vi "Check For Errors.vi"(8 "error in":errorcluster, 11 "Engine in":refnum<class "Engine.lvclass">) -> (0 "error out":errorcluster, 3 "Engine out":refnum<class "Engine.lvclass">)   [LabVIEW 2023, in "Engine.lvlib" / "Engine.lvclass"]
doc: "<b>Check for Errors </b>\n\nThis routine inspects the error code and generates a fault event if the value is non-zero (ie: a fault or warning is present)\n\nIt returns no error, ensuring that the software operates even if a fault is present."
uses:
  Library/Engine.lvclass
  Library/Engine.lvclass/Engine.ctl
  builds/Framework/Actor Framework.lvlibp/1abvi3w/vi.lib/ActorFramework/Actor/Read Actor Label.vi
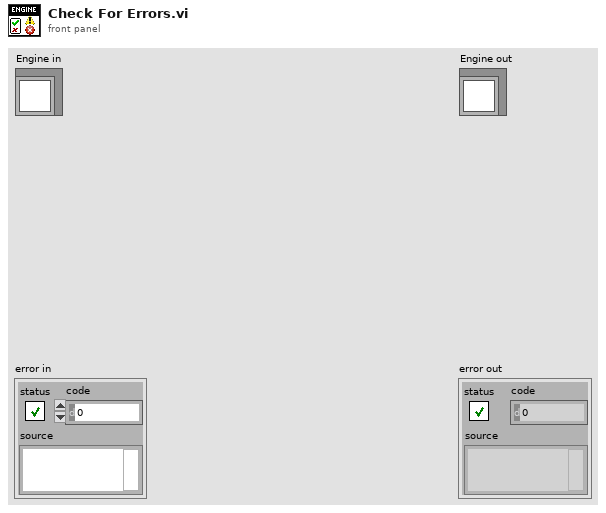
[diagram p1: front panel]
types:
  T1 = cluster{"Accessors:Actor Label":string, "error in":errorcluster}
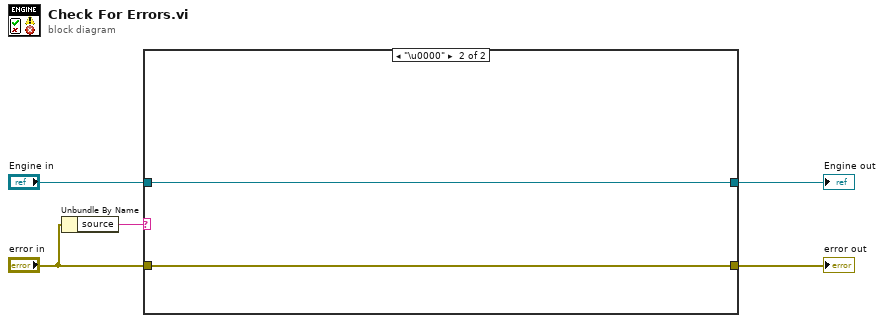
[diagram p0: block diagram]
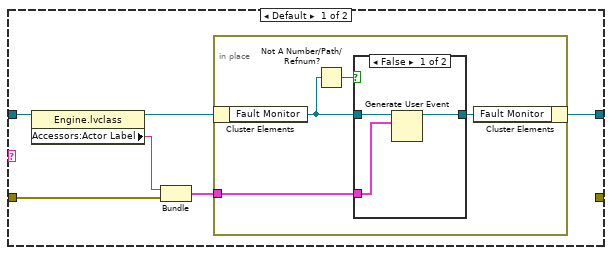
[diagram p2: hidden frame]
diagram:
  n1 = Unbundle By Name("error in") -> ("source"=w5:string)
  n2 = case shown="\"\"" w5 {
    tunnel: "Engine in" -> [w10 w21]
    tunnel: [w9 w21] -> w3
    tunnel: "error in" -> [w11 w20]
    tunnel: [_ w20] -> w1
    frame Default {
      n3 = property class="Engine.lvclass"(reference=w10) -> (reference out=w7:refnum<class "Engine.lvclass">, "Accessors:Actor Label"=w6:string)  [unwired: 1 in, 1 out]
      n4 = Bundle("Accessors:Actor Label"=w6, "error in"=w11) -> (w8:T1)  [unwired: 1 in]
      n5 = in-place {
        in-place-border: w8 -> [w12]
        n6 = in-place-cluster #1(w7) -> ("Fault Monitor"=w13:refnum<user-event>)
        n7 = Not A Number/Path/Refnum?(number/path/refnum=w13) -> (NaN/Path/Refnum?=w14:bool)
        n8 = case shown="False" w14 {
          tunnel: w13 -> [w18 w19]
          tunnel: [w17 w19] -> w15
          tunnel: w12 -> [w16 _]
          frame False {
            n9 = Generate User Event(user event=w18, event data cluster=w16) -> (user event out=w17:refnum<user-event>)  [unwired: 2 in, 1 out]
          }
          frame True {
          }
        }
        n10 = in-place-cluster #1("Fault Monitor"=w15) -> (w9:refnum<class "Engine.lvclass">)
      }
    }
    frame "\u0000" {
    }
  }
  "error out" <- w1
  "Engine out" <- w3
